vi "Set BER Floor.vi"(8 "error in":errorcluster, 10 "BER floor":dbl, 11 "eye scan in":refnum<class "niHighSpeedSerial Eye Scan v1 Host.lvclass">) -> (0 "error out":errorcluster, 3 "eye scan out":refnum<class "niHighSpeedSerial Eye Scan v1 Host.lvclass">)   [LabVIEW 2015, in "niHighSpeedSerial Eye Scan v1 Host.lvclass"]
doc: "Sets the BER Floor to be used for Eye Scan.\nNote that because it must be converted to a discrete prescale value, the actual BER Floor may be smaller than that requested.\nYou may see the coerced BER Floor by reading this property.\n\n<B>Input Parameters</B>\n\n<B>error in</B> describes error conditions that occur before this node runs. This input provides standard 'error in' functionality.\n\n<B>BER floor</B> is the minimum Bit Error Rate which may be computed.\n\n<B>eye scan in</B> Takes in a reference to your session from the previous VI.\n\n<B>Output Parameters</B>\n\n<B>error out</B> contains error information. This output provides standard 'error out' functionality.\n\n<B>eye scan out</B> passes a reference to your session to the next VI."
uses:
  <instrlib>/niHighSpeedSerial/Eye Scan/v1/Host/Eye Scan/niHighSpeedSerial Eye Scan v1 Host.lvclass
  <instrlib>/niHighSpeedSerial/Eye Scan/v1/Host/Eye Scan/niHighSpeedSerial Eye Scan v1 Host.lvclass/niHighSpeedSerial Eye Scan v1 Host.ctl
  <vilib>/Utility/error.llb/Error Cluster From Error Code.vi
  <vilib>/ErrorRing/Error Ring.xnode
  <instrlib>/niHighSpeedSerial/Eye Scan/v1/Host/Common/niHighSpeedSerial Eye Scan Common v1 Host.lvlib
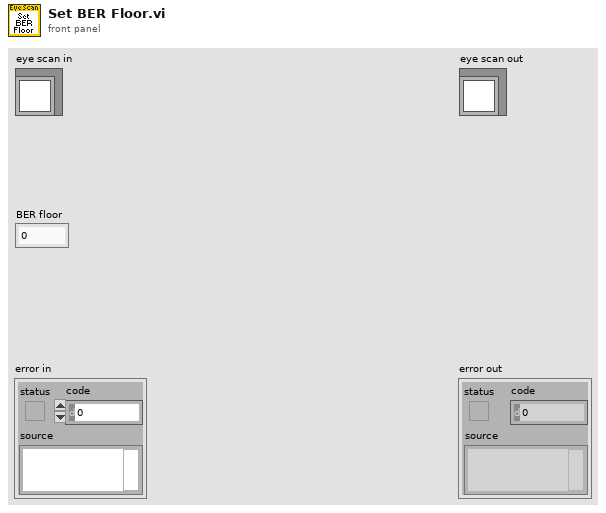
[diagram p1: front panel]
types:
  T1 = typedef "niHighSpeedSerial Eye Scan v1 Host.lvclass/Private Data.ctl" = cluster{"instruction target":refnum<class "niInstr Instruction Target v1 Host.lvclass">, "channels":T2[], "measure state":T3, "rx output divider":T4, "equalization mode":T5, "rx internal data width":T6, "BER floor":dbl, "number of points completed":i32, "rx output divider configured?":bool, "equalization mode configured?":bool, "rx data width configured?":bool}
  T2 = typedef "niHighSpeedSerial Eye Scan v1 Host.lvclass/Channel Data.ctl" = cluster{"instance":u8, "channel":refnum<class "niHighSpeedSerial Eye Scan Single Point v1 Host.lvclass">, "point iterator":refnum<class "niHighSpeedSerial Eye Scan Point Iterator v1 Host.lvclass">}
  T3 = typedef "niHighSpeedSerial Eye Scan v1 Host.lvclass/Measure State.ctl" = enum16{"Uninitialized", "Initialized", "Ready", "Measuring", "Finished", "Aborted"}
  T4 = typedef "niHighSpeedSerial Eye Scan Common v1 Host.lvlib/RX Output Divider.ctl" = enum16{"1", "2", "4", "8", "16"}
  T5 = typedef "niHighSpeedSerial Eye Scan Common v1 Host.lvlib/Equalization Mode.ctl" = enum16{"DFE", "LPM"}
  T6 = typedef "niHighSpeedSerial Eye Scan Common v1 Host.lvlib/Data Width.ctl" = enum16{"16 Bit", "20 Bit", "32 Bit", "40 Bit"}
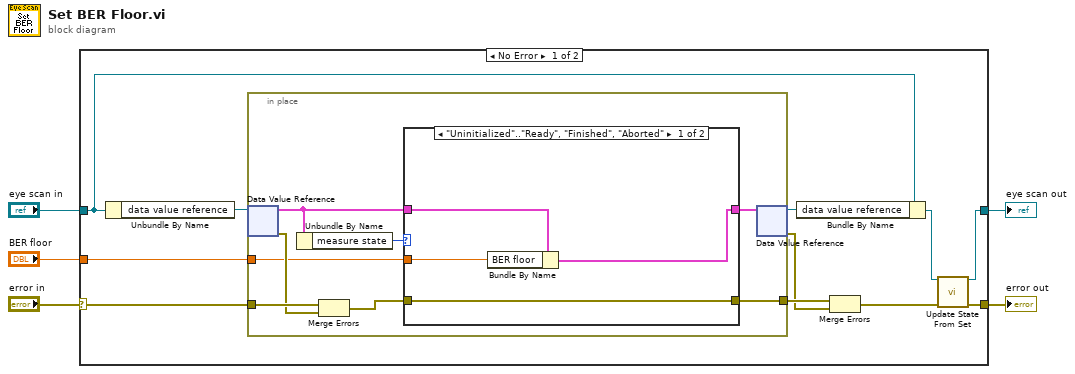
[diagram p0: block diagram]
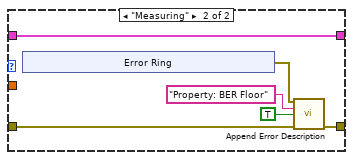
[diagram p2: hidden frame]
diagram:
  n1 = case shown="No Error" "error in" {
    selector: "error in" -> [w10 w40]
    tunnel: [w7 w40] -> w4
    tunnel: [w6 w39] -> w2
    tunnel: "eye scan in" -> [w14 w39]
    tunnel: "BER floor" -> [w13 _]
    frame No Error {
      n2 = Unbundle By Name(w14) -> ("data value reference"=w16:refnum<data-value>)
      n3 = in-place {
        in-place-border: w13 -> [w21]
        in-place-border: [w17] -> w12
        in-place-border: w10 -> [w24]
        n4 = in-place-dvr #1(w16) -> (w19:T1, w23:errorcluster)
        n5 = Unbundle By Name(w19) -> ("measure state"=w22:T3)
        n6 = Merge Errors(w24, w23) -> (w18:errorcluster)
        n7 = case shown="\"Uninitialized\"..\"Ready\", \"Finished\", \"Aborted\"" w22 {
          tunnel: w21 -> [w28 _]
          tunnel: [w27 w34] -> w20
          tunnel: w19 -> [w26 w34]
          tunnel: w18 -> [w25 w32]
          tunnel: [w25 w31] -> w17
          frame "Uninitialized".."Ready", "Finished", "Aborted" {
            n8 = Bundle By Name(cluster=w26, "BER floor"=w28) -> (w27:T1)
          }
          frame "Measuring" {
            n9 = xnode "Error Ring"() -> ("error out"=w33:errorcluster)
            n10 = call <instrlib>:"Append Error Description.vi"("error to append"=w33, "append string (\"\")"="Property: BER Floor" ("append string (\"\")"), "generate error?"=TRUE, "error in"=w32) -> ("error out"=w31:errorcluster)  [unwired: 11 in]
          }
        }
        n11 = in-place-dvr #1(w20) -> (w15:refnum<data-value>, w11:errorcluster)
      }
      n12 = Bundle By Name(cluster=w14, "data value reference"=w15) -> (w9:refnum<class "niHighSpeedSerial Eye Scan v1 Host.lvclass">)
      n13 = Merge Errors(w12, w11) -> (w8:errorcluster)
      n14 = call-dynamic "Update State From Set.vi"("eye scan in"=w9, "error in"=w8) -> ("eye scan out"=w6:refnum<class "niHighSpeedSerial Eye Scan v1 Host.lvclass">, "error out"=w7:errorcluster)  [unwired: 12 in]
    }
    frame Error {
    }
  }
  "error out" <- w4
  "eye scan out" <- w2
